vi "_032.vi"() -> ()   [LabVIEW 2024]
panel:
  out "Min Val":dbl
  out "Max Val":dbl
  in  "Array":dbl[](array[numeric])
  # "To find Max and Min Val with using Array :"
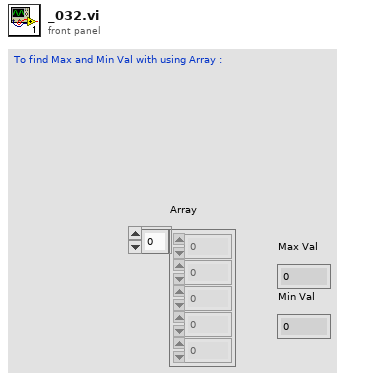
[diagram p1: front panel]
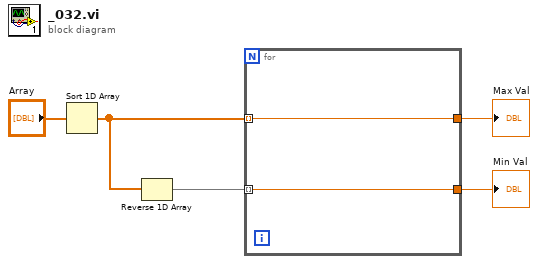
[diagram p0: block diagram]
diagram:
  n1 = Sort 1D Array(array="Array") -> (sorted array=w3:dbl[])
  n2 = Reverse 1D Array(array=w3) -> (reversed array=w2:dbl[])
  n3 = for {
    tunnel: [w7] -> w4
    tunnel: w3 -> [w7] mode=indexing
    tunnel: [w6] -> w1
    tunnel: w2 -> [w6] mode=indexing
  }
  "Max Val" <- w4
  "Min Val" <- w1
